vi "Memory.Pointer.Numeric.Count to Size.vi"(8 "error in (no error)":errorcluster, 10 "count":u64, 11 "Numeric Pointer in":refnum<class "Memory.Pointer.Numeric.lvclass">) -> (0 "error out":errorcluster, 2 "size":u64 format="%d bytes", 3 "Numeric Pointer out":refnum<class "Memory.Pointer.Numeric.lvclass">)   [LabVIEW 2016, in "LabVIEW Memory Manager.lvlib" / "Memory.Pointer.Numeric.lvclass"]
uses:
  Memory.Pointer.Numeric.lvclass
  Memory.Pointer.Numeric.lvclass/Memory.Pointer.Numeric.ctl
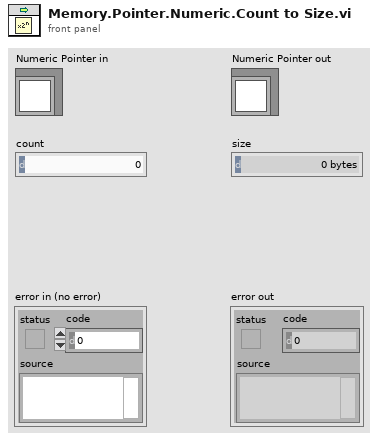
[diagram p1: front panel]
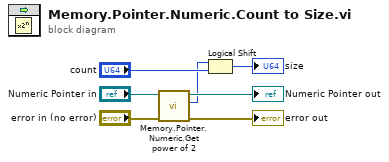
[diagram p0: block diagram]
diagram:
  n1 = call "Memory.Pointer.Numeric.Get power of 2.vi"("error in (no error)"="error in (no error)", "Memory.Pointer.Numeric in"="Numeric Pointer in") -> ("error out"=→"error out":errorcluster, "power of 2"=w2:i16, "Memory.Pointer.Numeric out"=→"Numeric Pointer out":refnum<class "Memory.Pointer.Numeric.lvclass">)  [unwired: 7 in]
  n2 = Logical Shift(y=w2, x="count") -> (x << y=→"size":u64)
